vi "motorFunctionWithReadout.vi"(0 "VISA Refnum in":refnum<visa-resource-name>, 1 "Fans":i32, 2 "zone 3 co2":dbl, 3 "zone 2 return":dbl, 4 "Light 1":i32, 5 "zone 2 co2":dbl, 6 "Light 3":i32, 7 "error in (no error)":errorcluster, 8 "zone 2 inlet":dbl, 9 "zone 3 inlet":dbl, 10 "zone 1 co2":dbl, 11 "Light in":i32, 12 "zone 1 return":dbl, 13 "zone 3 return":dbl, 14 "zone 1 inlet":dbl, 16 "fresh air":dbl) -> (18 "String":string, 20 "VISA Refnum out":refnum<visa-resource-name>, 27 "error out":errorcluster)   [LabVIEW 2019]
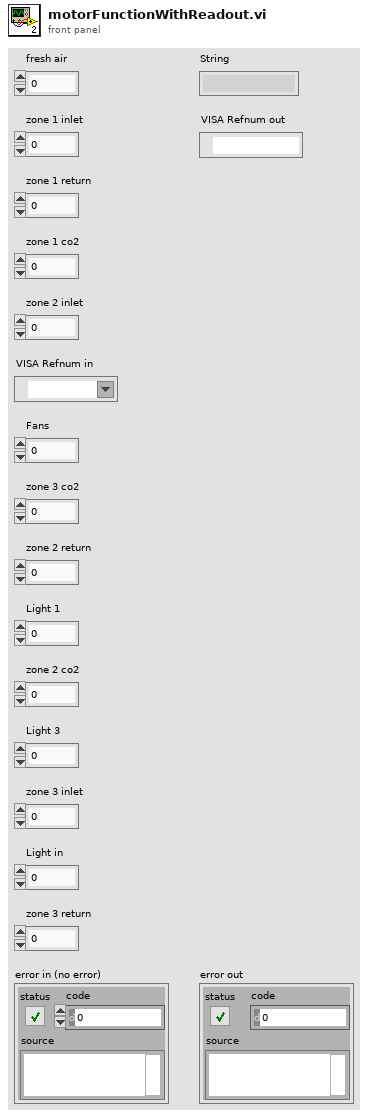
[diagram p1: front panel]
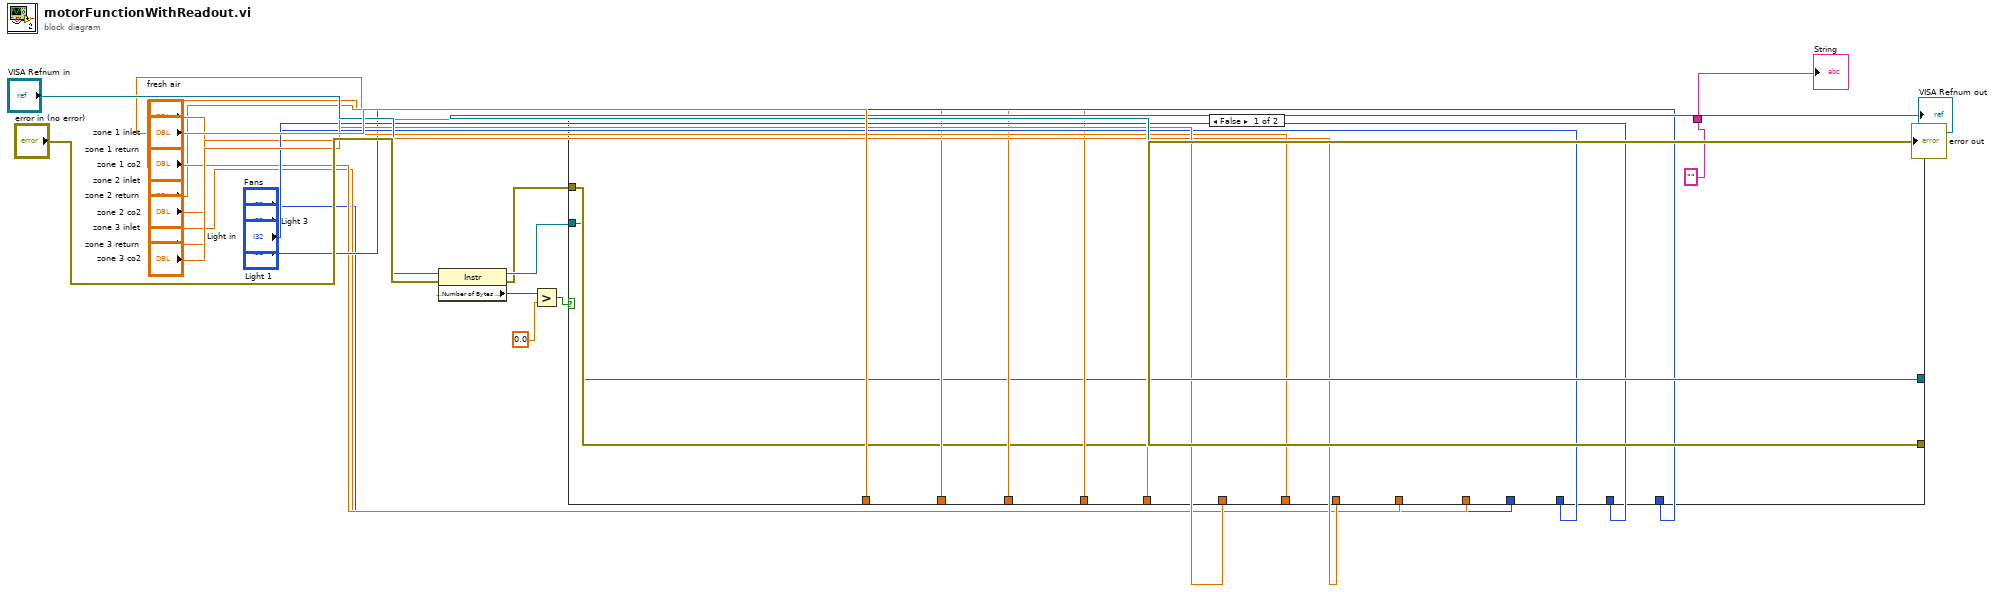
[diagram p0: block diagram]
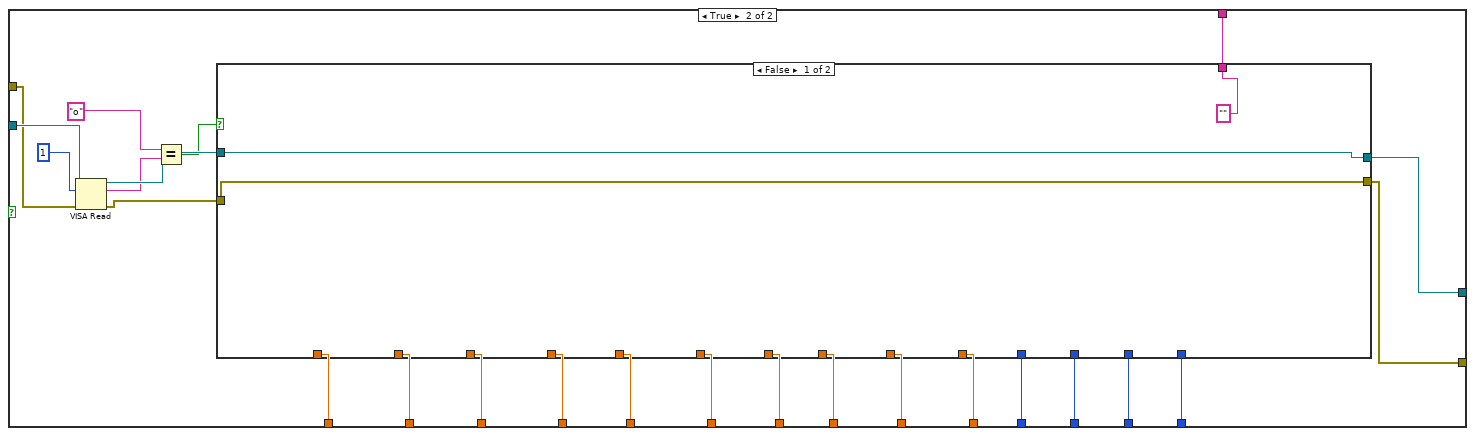
[diagram p2: hidden frame]
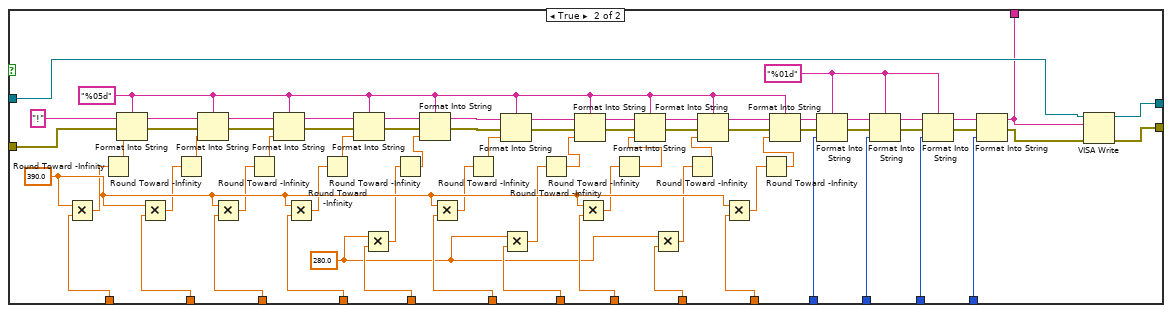
[diagram p3: hidden frame]
diagram:
  n1 = property class="Instr"(reference="VISA Refnum in", error in="error in (no error)") -> (reference out=w20:refnum<visa-resource-name>, error out=w19:errorcluster, "Serial Settings:Number of Bytes at Serial Port"=w22:u32)
  n2 = Greater?(x=w22, y=0.0) -> (0:w21:bool)
  n3 = case shown="False" w21 {
    tunnel: [w26 w51] -> w16
    tunnel: [w27 w50] -> w17
    tunnel: "Light 1" -> [_ w47]
    tunnel: "Light in" -> [_ w46]
    tunnel: "Light 3" -> [_ w45]
    tunnel: "Fans" -> [_ w44]
    tunnel: "zone 3 inlet" -> [_ w43]
    tunnel: "zone 1 co2" -> [_ w42]
    tunnel: "fresh air" -> [_ w41]
    tunnel: "zone 2 co2" -> [_ w40]
    tunnel: "zone 3 return" -> [_ w39]
    tunnel: "zone 3 co2" -> [_ w38]
    tunnel: "zone 2 return" -> [_ w37]
    tunnel: "zone 2 inlet" -> [_ w36]
    tunnel: "zone 1 inlet" -> [_ w32]
    tunnel: "zone 1 return" -> [_ w31]
    tunnel: w20 -> [w26 w30]
    tunnel: w19 -> [w27 w29]
    tunnel: ["" ("String") w28] -> w24
    frame False {
    }
    frame True {
      n4 = VISA Read(VISA resource name=w30, byte count=u32 1, error in (no error)=w29) -> (VISA resource name out=w52:refnum<visa-resource-name>, read buffer=w34:string, error out=w49:errorcluster)  [unwired: 1 out]
      n5 = Equal?(x="o" ("y"), y=w34) -> (x = y?=w48:bool)
      n6 = case shown="False" w48 {
        tunnel: [w54 w111] -> w51
        tunnel: [w55 w110] -> w50
        tunnel: w32 -> [_ w88]
        tunnel: w31 -> [_ w87]
        tunnel: w36 -> [_ w86]
        tunnel: w37 -> [_ w85]
        tunnel: w38 -> [_ w84]
        tunnel: w39 -> [_ w83]
        tunnel: w40 -> [_ w82]
        tunnel: w41 -> [_ w81]
        tunnel: w42 -> [_ w80]
        tunnel: w43 -> [_ w79]
        tunnel: w44 -> [_ w94]
        tunnel: w45 -> [_ w93]
        tunnel: w46 -> [_ w92]
        tunnel: w47 -> [_ w91]
        tunnel: w49 -> [w55 w90]
        tunnel: w52 -> [w54 w89]
        tunnel: ["" ("String") w56] -> w28
        frame False {
        }
        frame True {
          w57 = 280.0 ("x")
          w78 = 390.0 ("y")
          w98 = "%01d" ("format string")
          w105 = "%05d" ("format string")
          n7 = Multiply(x=w78, y=w88) -> (x*y=w58:dbl)
          n8 = Round Toward -Infinity(1:w58) -> (0:w77:dbl)
          n9 = Format Into String(format string=w105, initial string="!" ("write buffer"), error in=w90, w77) -> (resulting string=w125:string, error out=w126:errorcluster)
          n10 = Multiply(x=w78, y=w87) -> (x*y=w59:dbl)
          n11 = Round Toward -Infinity(1:w59) -> (0:w76:dbl)
          n12 = Format Into String(format string=w105, initial string=w125, error in=w126, w76) -> (resulting string=w123:string, error out=w124:errorcluster)
          n13 = Multiply(x=w78, y=w86) -> (x*y=w60:dbl)
          n14 = Round Toward -Infinity(1:w60) -> (0:w75:dbl)
          n15 = Format Into String(format string=w105, initial string=w123, error in=w124, w75) -> (resulting string=w121:string, error out=w122:errorcluster)
          n16 = Multiply(x=w78, y=w85) -> (x*y=w61:dbl)
          n17 = Round Toward -Infinity(1:w61) -> (0:w74:dbl)
          n18 = Format Into String(format string=w105, initial string=w121, error in=w122, w74) -> (resulting string=w119:string, error out=w120:errorcluster)
          n19 = Multiply(x=w57, y=w84) -> (x*y=w62:dbl)
          n20 = Round Toward -Infinity(1:w62) -> (0:w73:dbl)
          n21 = Format Into String(format string=w105, initial string=w119, error in=w120, w73) -> (resulting string=w117:string, error out=w118:errorcluster)
          n22 = Multiply(x=w78, y=w83) -> (x*y=w63:dbl)
          n23 = Round Toward -Infinity(1:w63) -> (0:w72:dbl)
          n24 = Format Into String(format string=w105, initial string=w117, error in=w118, w72) -> (resulting string=w115:string, error out=w116:errorcluster)
          n25 = Multiply(x=w57, y=w82) -> (x*y=w64:dbl)
          n26 = Round Toward -Infinity(1:w64) -> (0:w71:dbl)
          n27 = Format Into String(format string=w105, initial string=w115, error in=w116, w71) -> (resulting string=w114:string, error out=w113:errorcluster)
          n28 = Multiply(x=w78, y=w81) -> (x*y=w65:dbl)
          n29 = Round Toward -Infinity(1:w65) -> (0:w70:dbl)
          n30 = Format Into String(format string=w105, initial string=w114, error in=w113, w70) -> (resulting string=w107:string, error out=w109:errorcluster)
          n31 = Multiply(x=w57, y=w80) -> (x*y=w66:dbl)
          n32 = Round Toward -Infinity(1:w66) -> (0:w69:dbl)
          n33 = Format Into String(format string=w105, initial string=w107, error in=w109, w69) -> (resulting string=w106:string, error out=w108:errorcluster)
          n34 = Multiply(x=w78, y=w79) -> (x*y=w67:dbl)
          n35 = Round Toward -Infinity(1:w67) -> (0:w68:dbl)
          n36 = Format Into String(format string=w105, initial string=w106, error in=w108, w68) -> (resulting string=w101:string, error out=w104:errorcluster)
          n37 = Format Into String(format string=w98, initial string=w101, error in=w104, w94) -> (resulting string=w100:string, error out=w103:errorcluster)
          n38 = Format Into String(format string=w98, initial string=w100, error in=w103, w93) -> (resulting string=w99:string, error out=w102:errorcluster)
          n39 = Format Into String(format string=w98, initial string=w99, error in=w102, w92) -> (resulting string=w96:string, error out=w97:errorcluster)
          n40 = Format Into String(initial string=w96, error in=w97, w91) -> (resulting string=w56:string, error out=w95:errorcluster)  [unwired: 1 in]
          n41 = VISA Write(VISA resource name=w89, write buffer=w56, error in (no error)=w95) -> (VISA resource name out=w111:refnum<visa-resource-name>, error out=w110:errorcluster)  [unwired: 1 out]
        }
      }
    }
  }
  "String" <- w24
  "error out" <- w17
  "VISA Refnum out" <- w16
